vi "niDTS BT INSTR TX Fetch Results.vi"(8 "error in (no error)":errorcluster, 10 "ResultsIndex":u8=1, 11 "niDTS BT INSTR TX in":refnum<class "niDTS BT INSTR TX.lvclass">) -> (0 "error out":errorcluster, 2 "Results":T1 {"OBW Resutls"."Stop Frequency (Hz)" format="%#_4p"; "OBW Resutls"."Start Frequency (Hz)" format="%#_4p"}, 3 "niDTS BT INSTR TX out":refnum<class "niDTS BT INSTR TX.lvclass">)   [LabVIEW 2015, in "niDTS BT.lvlib" / "niDTS BT INSTR TX.lvclass"]
uses:
  niDTS BT INSTR TX.lvclass
  Tests/Tx Test/Includes/niDTS BT Tx Test INC Results.ctl
  Tests/Tx Test/Includes/niDTS BT Tx Test INC IBE Results.ctl
  Tests/Tx Test/Includes/niDTS BT Tx Test INC OBW Results.ctl
  Tests/Tx Test/Includes/niDTS BT Tx Test INC TXP Results.ctl
  Tests/Tx Test/Includes/niDTS BT Tx Test INC DEVM Results.ctl
  Tests/Tx Test/Includes/niDTS BT Tx Test INC CF Stability Results.ctl
  Tests/Tx Test/Includes/niDTS BT Tx Test INC CFO Resutls.ctl
  Tests/Tx Test/Includes/niDTS BT Tx Test INC Character Results.ctl
  niDTS BT.lvlib
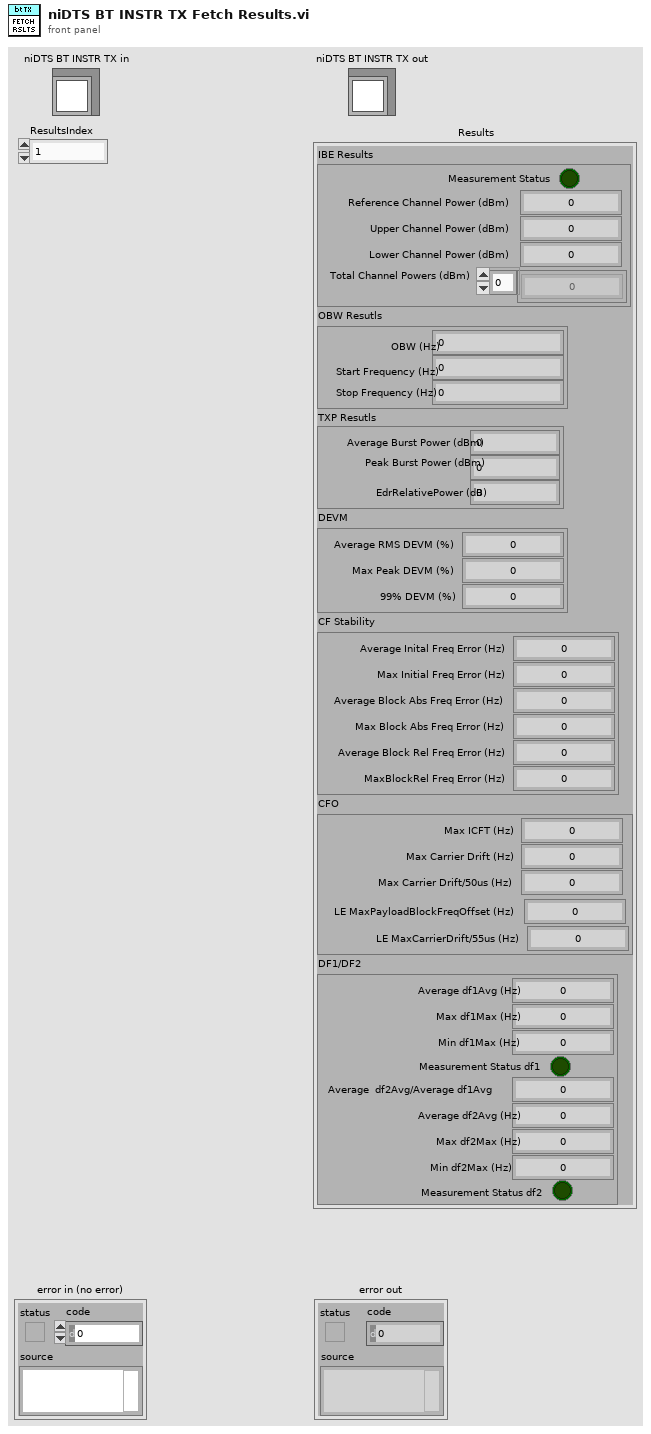
[diagram p1: front panel]
types:
  T1 = typedef "niDTS BT.lvlib/niDTS BT Tx Test INC Results.ctl" = cluster{"IBE Results":T2, "OBW Resutls":T3, "TXP Resutls":T4, "DEVM":T5, "CF Stability":T6, "CFO":T7, "DF1/DF2":T8}
  T2 = typedef "niDTS BT.lvlib/niDTS BT Tx Test INC IBE Results.ctl" = cluster{"Measurement Status":bool, "Reference Channel Power (dBm)":dbl, "Upper Channel Power (dBm)":dbl, "Lower Channel Power (dBm)":dbl, "Total Channel Powers (dBm)":dbl[]}
  T3 = typedef "niDTS BT.lvlib/niDTS BT Tx Test INC OBW Results.ctl" = cluster{"OBW (Hz)":dbl, "Start Frequency (Hz)":dbl, "Stop Frequency (Hz)":dbl}
  T4 = typedef "niDTS BT.lvlib/niDTS BT Tx Test INC TXP Results.ctl" = cluster{"Average Burst Power (dBm)":dbl, "Peak Burst Power (dBm)":dbl, "EdrRelativePower (dB)":dbl}
  T5 = typedef "niDTS BT.lvlib/niDTS BT Tx Test INC DEVM Results.ctl" = cluster{"Average RMS DEVM (%)":dbl, "Max Peak DEVM (%)":dbl, "99% DEVM (%)":dbl}
  T6 = typedef "niDTS BT.lvlib/niDTS BT Tx Test INC CF Stability Results.ctl" = cluster{"Average Inital Freq Error (Hz)":dbl, "Max Initial Freq Error (Hz)":dbl, "Average Block Abs Freq Error (Hz)":dbl, "Max Block Abs Freq Error (Hz)":dbl, "Average Block Rel Freq Error (Hz)":dbl, "MaxBlockRel Freq Error (Hz)":dbl}
  T7 = typedef "niDTS BT.lvlib/niDTS BT Tx Test INC CFO Resutls.ctl" = cluster{"Max ICFT (Hz)":dbl, "Max Carrier Drift (Hz)":dbl, "Max Carrier Drift/50us (Hz)":dbl, "LE MaxPayloadBlockFreqOffset (Hz)":dbl, "LE MaxCarrierDrift/55us (Hz)":dbl}
  T8 = typedef "niDTS BT.lvlib/niDTS BT Tx Test INC Character Results.ctl" = cluster{"Average df1Avg (Hz)":dbl, "Max df1Max (Hz)":dbl, "Min df1Max (Hz)":dbl, "Measurement Status df1":bool, "Average  df2Avg/Average df1Avg":dbl, "Average df2Avg (Hz)":dbl, "Max df2Max (Hz)":dbl, "Min df2Max (Hz)":dbl, "Measurement Status df2":bool}
  T9 = typedef "niDTS BT.lvlib/niDTS BT INSTR TX.lvclass/niDTS BT INSTR TX INC ModAcc Result.ctl" = cluster{"DEVM":T5, "CF Stability":T6, "CFO":T7, "DF1/DF2":T8}
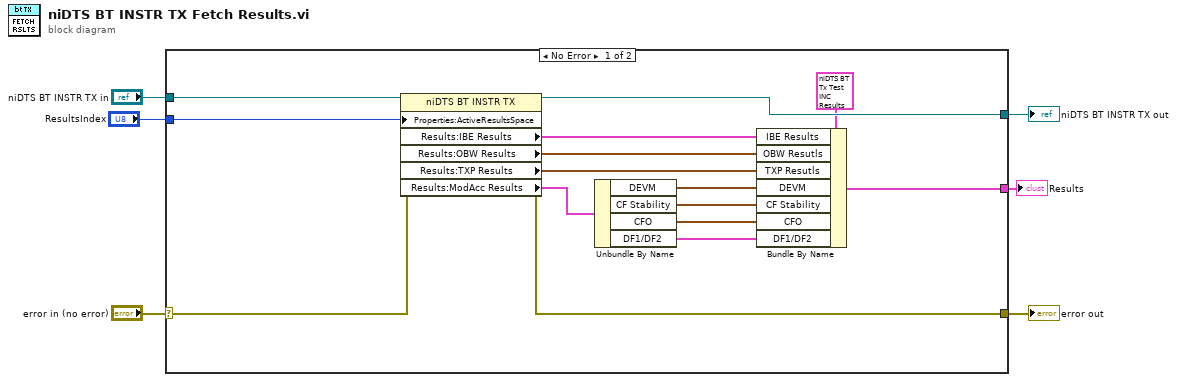
[diagram p0: block diagram]
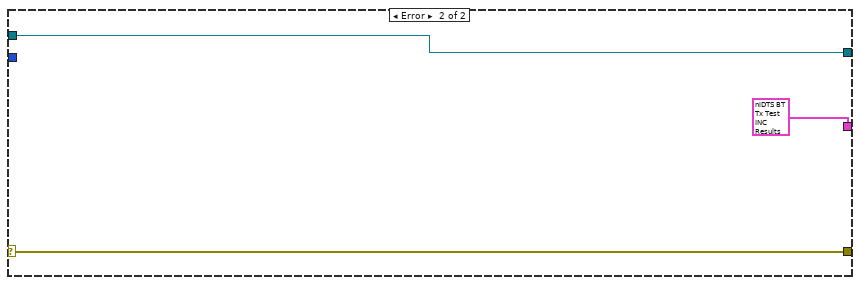
[diagram p2: hidden frame]
diagram:
  n1 = case shown="No Error" "error in (no error)" {
    selector: "error in (no error)" -> [w17 w24]
    tunnel: [w8 w24] -> w5
    tunnel: [w20 w23] -> w3
    tunnel: "niDTS BT INSTR TX in" -> [w21 w23]
    tunnel: [w9 T1 {"IBE Results"={"Measurement Status"=FALSE, "Reference Channel Power (dBm)"=0.0, "Upper Channel Power (dBm)"=0.0, "Lower Channel Power (dBm)"=0.0, "Total Channel Powers (dBm)"=[]}, "OBW Resutls"={"OBW (Hz)"=0.0, "Start Frequency (Hz)"=0.0, "Stop Frequency (Hz)"=0.0}, "TXP Resutls"={"Average Burst Power (dBm)"=0.0, "Peak Burst Power (dBm)"=0.0, "EdrRelativePower (dB)"=0.0}, "DEVM"={"Average RMS DEVM (%)"=0.0, "Max Peak DEVM (%)"=0.0, "99% DEVM (%)"=0.0}, "CF Stability"={"Average Inital Freq Error (Hz)"=0.0, "Max Initial Freq Error (Hz)"=0.0, "Average Block Abs Freq Error (Hz)"=0.0, "Max Block Abs Freq Error (Hz)"=0.0, "Average Block Rel Freq Error (Hz)"=0.0, "MaxBlockRel Freq Error (Hz)"=0.0}, "CFO"={"Max ICFT (Hz)"=0.0, "Max Carrier Drift (Hz)"=0.0, "Max Carrier Drift/50us (Hz)"=0.0, "LE MaxPayloadBlockFreqOffset (Hz)"=0.0, "LE MaxCarrierDrift/55us (Hz)"=0.0}, "DF1/DF2"={"Average df1Avg (Hz)"=0.0, "Max df1Max (Hz)"=0.0, "Min df1Max (Hz)"=0.0, "Measurement Status df1"=FALSE, "Average  df2Avg/Average df1Avg"=0.0, "Average df2Avg (Hz)"=0.0, "Max df2Max (Hz)"=0.0, "Min df2Max (Hz)"=0.0, "Measurement Status df2"=FALSE}} ("Results")] -> w2
    tunnel: "ResultsIndex" -> [w7 _]
    frame No Error {
      n2 = property class="niDTS BT INSTR TX"(reference=w21, error in=w17, "Properties:ActiveResultsSpace"=w7) -> (reference out=w20:refnum<class "niDTS BT INSTR TX.lvclass">, error out=w8:errorcluster, "Results:IBE Results"=w18:T2, "Results:OBW Results"=w16:T3, "Results:TXP Results"=w15:T4, "Results:ModAcc Results"=w14:T9)
      n3 = Unbundle By Name(w14) -> ("DEVM"=w13:T5, "CF Stability"=w12:T6, "CFO"=w11:T7, "DF1/DF2"=w10:T8)
      n4 = Bundle By Name(cluster=T1 {"IBE Results"={"Measurement Status"=FALSE, "Reference Channel Power (dBm)"=0.0, "Upper Channel Power (dBm)"=0.0, "Lower Channel Power (dBm)"=0.0, "Total Channel Powers (dBm)"=[]}, "OBW Resutls"={"OBW (Hz)"=0.0, "Start Frequency (Hz)"=0.0, "Stop Frequency (Hz)"=0.0}, "TXP Resutls"={"Average Burst Power (dBm)"=0.0, "Peak Burst Power (dBm)"=0.0, "EdrRelativePower (dB)"=0.0}, "DEVM"={"Average RMS DEVM (%)"=0.0, "Max Peak DEVM (%)"=0.0, "99% DEVM (%)"=0.0}, "CF Stability"={"Average Inital Freq Error (Hz)"=0.0, "Max Initial Freq Error (Hz)"=0.0, "Average Block Abs Freq Error (Hz)"=0.0, "Max Block Abs Freq Error (Hz)"=0.0, "Average Block Rel Freq Error (Hz)"=0.0, "MaxBlockRel Freq Error (Hz)"=0.0}, "CFO"={"Max ICFT (Hz)"=0.0, "Max Carrier Drift (Hz)"=0.0, "Max Carrier Drift/50us (Hz)"=0.0, "LE MaxPayloadBlockFreqOffset (Hz)"=0.0, "LE MaxCarrierDrift/55us (Hz)"=0.0}, "DF1/DF2"={"Average df1Avg (Hz)"=0.0, "Max df1Max (Hz)"=0.0, "Min df1Max (Hz)"=0.0, "Measurement Status df1"=FALSE, "Average  df2Avg/Average df1Avg"=0.0, "Average df2Avg (Hz)"=0.0, "Max df2Max (Hz)"=0.0, "Min df2Max (Hz)"=0.0, "Measurement Status df2"=FALSE}} ("Results"), "IBE Results"=w18, "OBW Resutls"=w16, "TXP Resutls"=w15, "DEVM"=w13, "CF Stability"=w12, "CFO"=w11, "DF1/DF2"=w10) -> (w9:T1)
    }
    frame Error {
    }
  }
  "error out" <- w5
  "niDTS BT INSTR TX out" <- w3
  "Results" <- w2
